vi "DAQ.Simulate Noisy AI.vi"(4 "Simulate Waveguide [T]":bool=TRUE, 6 "Waveguide Cluster":T1={"Vsource Index"=0, "Vsg Index"=1, "V+"=0, "V-"=0}, 8 "error in (no error)":errorcluster, 11 "Instrument.DAQ in":refnum<class "Instrument.DAQ.lvclass">) -> (0 "error out":errorcluster, 3 "Instrument.DAQ out":refnum<class "Instrument.DAQ.lvclass">)   [LabVIEW 2019, in "Instrument.DAQ.lvclass"]
uses:
  Instrument.DAQ.lvclass
  Waveguide Model/Waveguide Model--Cluster.ctl
  Instrument.DAQ.lvclass/Instrument.DAQ.ctl
  <vilib>/Analysis/2dsp.llb/Real FFT.vi
  <vilib>/Analysis/2dsp.llb/Inverse Real FFT.vi
  <vilib>/measure/NI_MABase.lvlib
  <vilib>/Analysis/NI_AALPro.lvlib
panel:
  in  "Noise Cluster":T2={"1/f vs. Uniform "=1.0, "60Hz Amplitude"=0.005, "Gauss/Unif %"=0.5, "Noise Amp"=0.005}
  out "Signal Graph":waveform(dbl)[](graph)
  out "Noisy Signal Graph":waveform(dbl)[](graph)
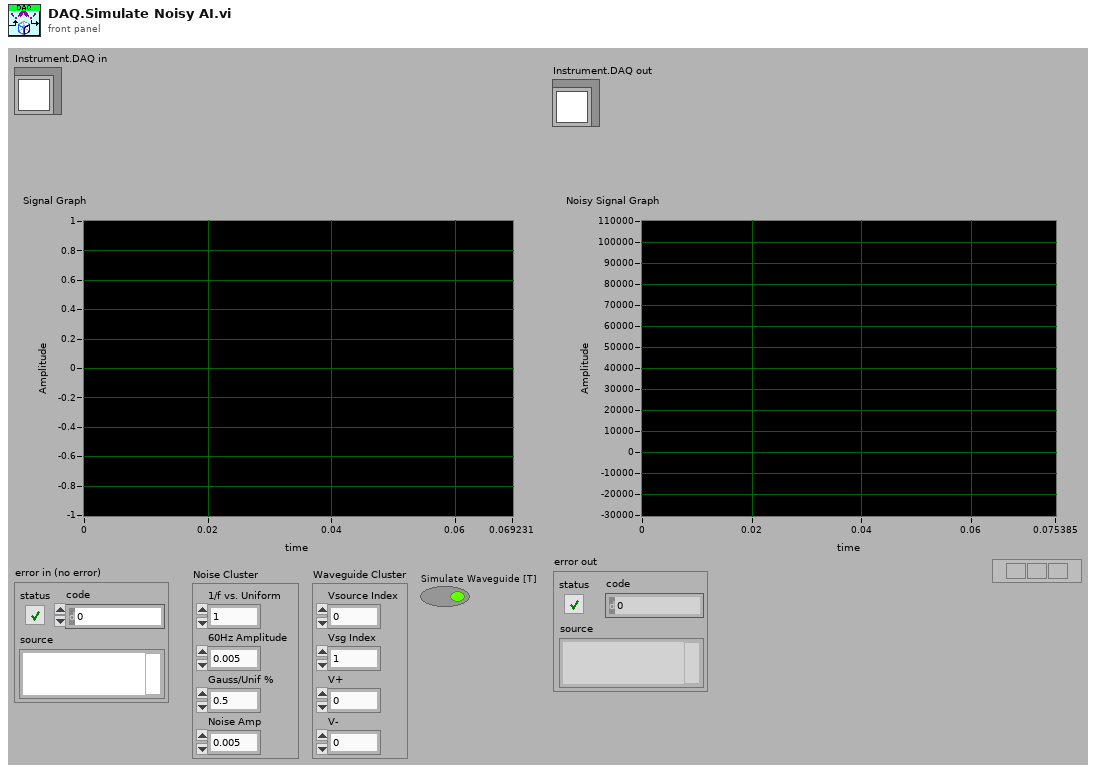
[diagram p1: front panel]
types:
  T1 = typedef "Instrument.DAQ.lvclass/Waveguide Model--Cluster.ctl" = cluster{"Vsource Index":i32, "Vsg Index":i32, "V+":i32, "V-":i32}
  T2 = cluster{"1/f vs. Uniform ":dbl, "60Hz Amplitude":dbl, "Gauss/Unif %":dbl, "Noise Amp":dbl}
  T3 = typedef "Instrument.DAQ.lvclass/Simulation Mode--enum.ctl" = enum16{"AI = HW simulated", "AI = noise*AO", "AI = waveguide"}
  T4 = typedef "Instrument.DAQ.lvclass/DAQ.Sampling.Sampling--Cluster.ctl" = cluster{"Fs":dbl, "#s":i32}
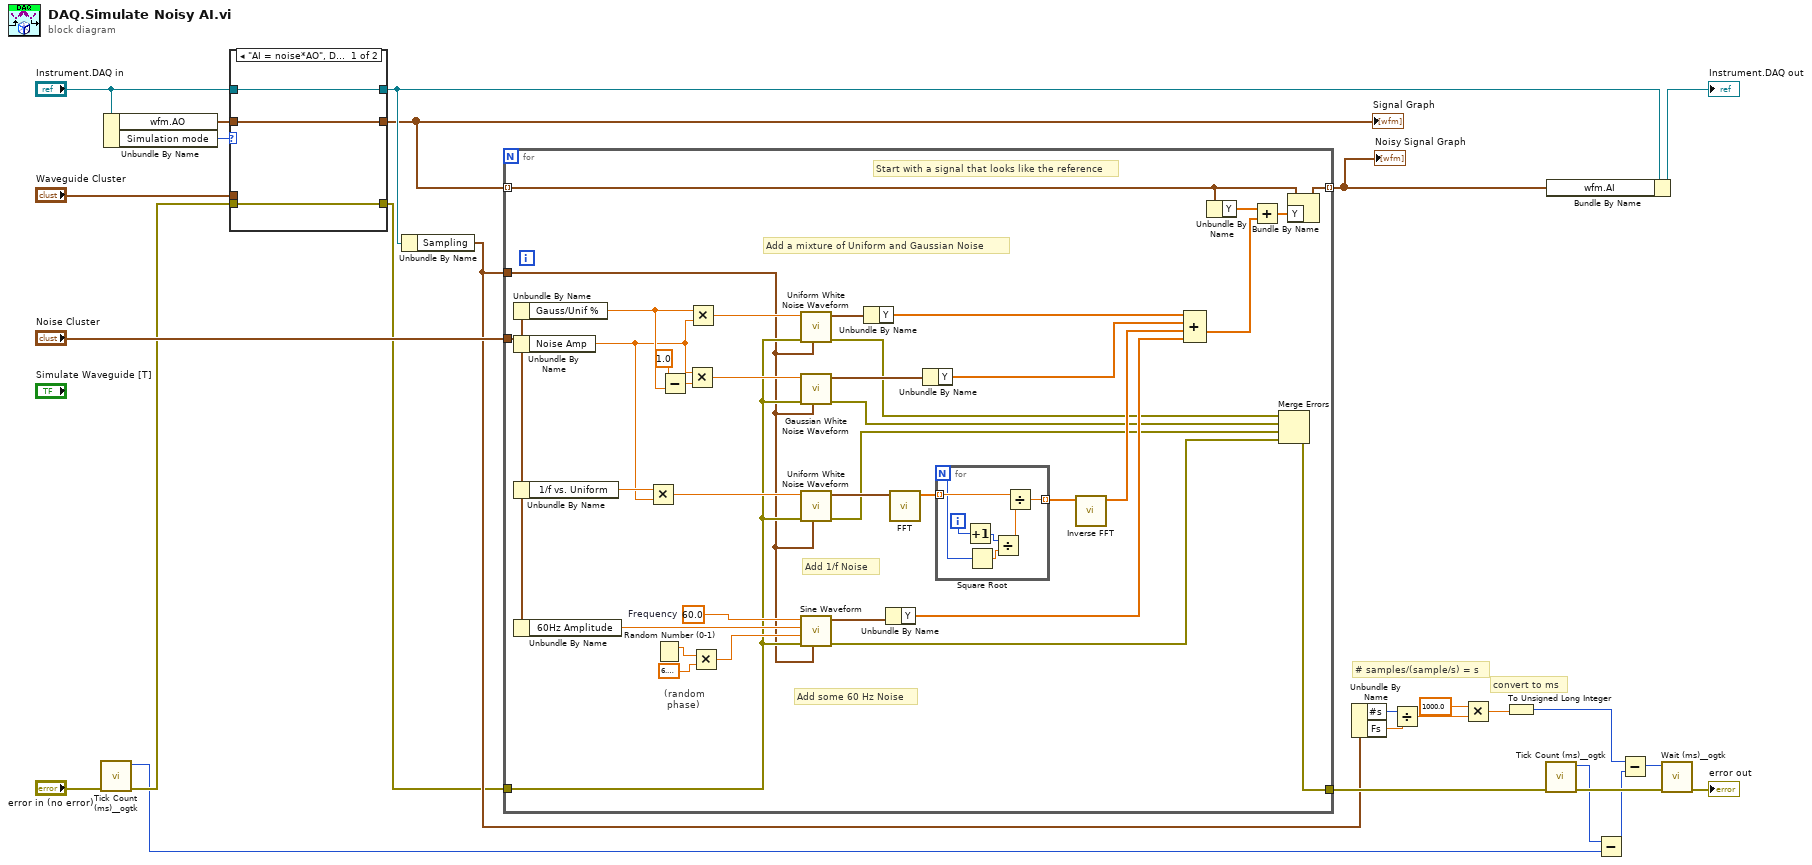
[diagram p0: block diagram]
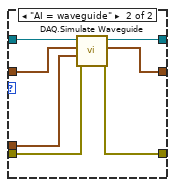
[diagram p2: hidden frame]
diagram:
  # "convert to ms"
  # "# samples/(sample/s) = s"
  n1 = call <userlib>:"Tick Count (ms)__ogtk.vi"("error in (no error)"="error in (no error)") -> ("error out"=w12:errorcluster, "millisecond timer value"=w9:u32)  [unwired: 9 in]
  n2 = Unbundle By Name("Instrument.DAQ in") -> ("wfm.AO"=w7:waveform(dbl)[], "Simulation mode"=w6:T3)
  n3 = case shown="\"AI = noise*AO\", Default" w6 {
    tunnel: w12 -> [w28 w32]
    tunnel: [w28 w31] -> w8
    tunnel: [w27 w36] -> w2
    tunnel: "Waveguide Cluster" -> [_ w30]
    tunnel: w7 -> [w27 w35]
    tunnel: "Instrument.DAQ in" -> [w29 w34]
    tunnel: [w29 w33] -> w4
    frame "AI = noise*AO", Default {
    }
    frame "AI = waveguide" {
      n4 = call "DAQ.Simulate Waveguide.vi"("error in (no error)"=w32, "Waveguide Cluster"=w30, "AO []"=w35, "Instrument.DAQ in"=w34) -> ("error out"=w31:errorcluster, "AI []"=w36:waveform(dbl)[], "Instrument.DAQ out"=w33:refnum<class "Instrument.DAQ.lvclass">)  [unwired: 5 in]
    }
  }
  "Signal Graph" <- w2
  n5 = Unbundle By Name(w4) -> ("Sampling"=w10:T4)
  n6 = for {
    tunnel: "Noise Cluster" -> [w52]
    tunnel: w10 -> [w42]
    tunnel: [w43] -> w1 mode=indexing
    tunnel: w8 -> [w46]
    tunnel: [w37] -> w25
    tunnel: w2 -> [w38] mode=indexing
    w47 = 60.0  # Frequency
    # "Start with a signal that looks like the reference"
    # "Add 1/f Noise"
    # "(random\n phase)"
    # "Add some 60 Hz Noise"
    # "Add a mixture of Uniform and Gaussian Noise"
    n7 = Unbundle By Name(w52) -> ("Gauss/Unif %"=w57:dbl)
    n8 = Unbundle By Name(w52) -> ("Noise Amp"=w39:dbl)
    n9 = Unbundle By Name(w52) -> ("1/f vs. Uniform"=w56:dbl)
    n10 = Unbundle By Name(w52) -> ("60Hz Amplitude"=w55:dbl)
    n11 = Multiply(x=w56, y=w39) -> (x*y=w63:dbl)
    n12 = Random Number (0-1)() -> (number: 0 to 1=w67:dbl)
    n13 = Subtract(x=1.0, y=w57) -> (x-y=w70:dbl)
    n14 = Multiply(x=w39, y=w70) -> (x*y=w51:dbl)
    n15 = Multiply(x=w57, y=w39) -> (x*y=w50:dbl)
    n16 = Multiply(x=w67, y=6.283185307179586) -> (x*y=w49:dbl)
    n17 = call <vilib>:"Uniform White Noise Waveform.vi"("sampling info"=w42, "error in (no error)"=w46, "amplitude"=w50) -> ("error out"=w40:errorcluster, "signal out"=w71:waveform(dbl))  [unwired: 7 in]
    n18 = call <vilib>:"Gaussian White Noise Waveform.vi"("sampling info"=w42, "error in (no error)"=w46, "standard deviation"=w51) -> ("error out"=w41:errorcluster, "signal out"=w72:waveform(dbl))  [unwired: 7 in]
    n19 = call <vilib>:"Uniform White Noise Waveform.vi"("sampling info"=w42, "error in (no error)"=w46, "amplitude"=w63) -> ("error out"=w45:errorcluster, "signal out"=w62:waveform(dbl))  [unwired: 7 in]
    n20 = call <vilib>:"Sine Waveform.vi"("sampling info"=w42, "error in (no error)"=w46, "phase"=w49, "amplitude"=w55, "frequency"=w47) -> ("error out"=w44:errorcluster, "signal out"=w66:waveform(dbl))  [unwired: 5 in]
    n21 = Unbundle By Name(w71) -> ("Y"=w65:dbl[])
    n22 = Unbundle By Name(w66) -> ("Y"=w61:dbl[])
    n23 = call-poly <vilib>:"FFT.vi"("X"=w62) -> ("FFT {X}"=w48:cdb[])  [unwired: 9 in, 1 out]
    n24 = Unbundle By Name(w72) -> ("Y"=w58:dbl[])
    n25 = for {
      N -> [w76]
      tunnel: [w79] -> w64 mode=indexing
      tunnel: w48 -> [w78] mode=indexing
      i -> [w77]
      n26 = Increment(x=w77) -> (x+1=w74:i32)
      n27 = Square Root(x=w76) -> (sqrt(x)=w75:dbl)
      n28 = Divide(x=w74, y=w75) -> (x/y=w73:dbl)
      n29 = Divide(x=w78, y=w73) -> (x/y=w79:cdb)
    }
    n30 = call-poly <vilib>:"Inverse FFT.vi"("FFT {X}"=w64) -> ("X"=w60:dbl[])  [unwired: 9 in, 1 out]
    n31 = Compound Arithmetic op=ADD(w65, w58, w60, w61) -> (w59:dbl[])
    n32 = Unbundle By Name(w38) -> ("Y"=w54:dbl[])
    n33 = Add(x=w54, y=w59) -> (x+y=w53:dbl[])
    n34 = Merge Errors(w40, w41, w45, w44) -> (w37:errorcluster)
    n35 = Bundle By Name(cluster=w38, "Y"=w53) -> (w43:waveform(dbl))
  }
  "Noisy Signal Graph" <- w1
  n36 = Unbundle By Name(w10) -> ("#s"=w15:i32, "Fs"=w16:dbl)
  n37 = Divide(x=w15, y=w16) -> (x/y=w19:dbl)
  n38 = Multiply(x=1000.0, y=w19) -> (x*y=w18:dbl)
  n39 = To Unsigned Long Integer(number=w18) -> (unsigned 32bit integer=w14:u32)
  n40 = call <userlib>:"Tick Count (ms)__ogtk.vi"("error in (no error)"=w25) -> ("error out"=w24:errorcluster, "millisecond timer value"=w20:u32)  [unwired: 9 in]
  n41 = Bundle By Name(cluster=w4, "wfm.AI"=w1) -> (→"Instrument.DAQ out":refnum<class "Instrument.DAQ.lvclass">)
  n42 = Subtract(x=w20, y=w9) -> (x-y=w21:u32)
  n43 = Subtract(x=w14, y=w21) -> (x-y=w22:u32)
  n44 = call <userlib>:"Wait (ms)__ogtk.vi"("error in (no error)"=w24, "milliseconds to wait"=w22) -> ("error out"=→"error out":errorcluster)  [unwired: 8 in, 1 out]
